vi "dfd_Create XML String for Subband Filters.vi"(7 "Bank":enum16{"AnalysisBank", "SynthesisBank"}(ring), 11 "filters":T1[](array[typedef]) {"mMRate_SumWl" min=1 max=32 step=1; "mMRate_InputIwl" min=1 max=32 step=1; "mMRate_GainWl" min=1 max=32 step=1; "mMRate_OutputWl" min=1 max=32 step=1; "mMRate_InputWl" min=1 max=32 step=1; "mMRate_CoefWl" min=1 max=32 step=1; "mMRate_Mode" items=["Default"=-1, "No Rate Change"=0, "Interpolation"=1, "Decimation"=2, "Interpolated"=3, "Rational"=4]}) -> (3 "xml string out":string)   [LabVIEW 2017, in "NI_DigFilter_FilterBank.lvlib"]
uses:
  <vilib>/addons/Digital Filter Design/NI_DigFilter_FilterBank.lvlib
  <vilib>/addons/Digital Filter Design/_Objects.llb/DFD Multirate Filter Obj.ctl
  <vilib>/addons/Digital Filter Design/_Objects.llb/DFD Multirate Mode.ctl
  <vilib>/addons/Digital Filter Design/_Objects.llb/DFD Coef Norm Type.ctl
  <vilib>/addons/Digital Filter Design/_Objects.llb/DFD Round-off Mode.ctl
  <vilib>/addons/Digital Filter Design/_Objects.llb/DFD FXP MRate Multiply Mode.ctl
  <vilib>/addons/Digital Filter Design/NI_DigFilter_Process.lvlib
  <vilib>/addons/Digital Filter Design/NI_DigFilterLicensed.lvlib
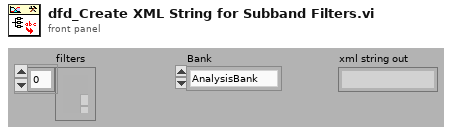
[diagram p1: front panel]
types:
  T1 = typedef "NI_DigFilterLicensed.lvlib/DFD Multirate Filter Obj.ctl" = cluster{"mMRate_Structure":enum16{"CIC", "FIR", "IIR", "Lattice"}, "mMRate_Mode":T2, "mMRate_Factor":i32, "mMRate_FIRParams":cluster{"mMRate_FIR_H":dbl[], "mMRate_FIR_IsNyquist?":bool, "mMRate_FIR_IsSymmetric?":bool}, "mMRate_CICParams":cluster{"mMRate_CIC_#Stage":i32, "mMRate_CIC_Lag":i32, "mMRate_CIC_Type":enum16{"Lowpass", "Highpass"}}, "mMRate_Order":i32, "mMRate_Version":string, "mMRate_Comments":string, "mMRate_RationalFactor":cluster{"mMRate_L":i32, "mMRate_M":i32}, "mMRate_Fs":dbl, "mMRate_Quantized?":bool, "mMRate_QFilterGain":dbl, "mMRate_CoefWl":i16, "mMRate_Scaling":cluster{"mMRate_ScaleByPowerOf2?":bool, "mMRate_ScaleType":T3}, "mMRate_InputWl":i16, "mMRate_OutputWl":i16, "mMRate_OutputMode":T4, "mMRate_MultMode":T5, "mMRate_BitPruning":bool, "mMRate_GainWl":i16, "mMRate_OutputFwl":i16, "mMRate_SumIwl":i16, "mMRate_InputIwl ":i16, "mMRate_SumWl":i16, "mMRate_CoefIwl":i16}
  T2 = typedef "NI_DigFilterLicensed.lvlib/DFD Multirate Mode.ctl" = i16
  T3 = typedef "NI_DigFilterLicensed.lvlib/DFD Coef Norm Type.ctl" = enum16{"No Norm", "Time Domain 1-Norm", "Time Domain 2-Norm", "Time Domain Inf-Norm"}
  T4 = typedef "NI_DigFilterLicensed.lvlib/DFD Round-off Mode.ctl" = enum16{"Nearest", "Truncation"}
  T5 = typedef "NI_DigFilterLicensed.lvlib/DFD FXP MRate Multiply Mode.ctl" = enum16{"Truncated", "Full"}
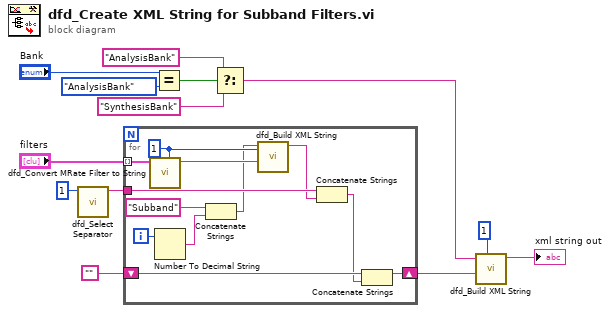
[diagram p0: block diagram]
diagram:
  n1 = call <vilib>:"dfd_Select Separator.vi"("indent order"=1) -> ("separator"=w11:string)  [unwired: 10 out]
  n2 = for {
    tunnel: "filters" -> [w25] mode=indexing
    tunnel: w11 -> [w24]
    shift-right: [w15] -> w12
    shift-left: "" -> [w16]
    i -> [w23]
    w22 = 1 ("indent order")
    n3 = call <vilib>:"dfd_Convert MRate Filter to String.vi"("indent order"=w22, "multirate filter in"=w25) -> ("xml string"=w20:string)  [unwired: 1 in, 8 out]
    n4 = Number To Decimal String(number=w23) -> (decimal integer string=w18:string)  [unwired: 1 out]
    n5 = Concatenate Strings("Subband" ("string"), w18) -> (w17:string)
    n6 = call <vilib>:"dfd_Build XML String.vi"("indent order"=w22, "string in"=w20, "element name"=w17) -> ("xml string out"=w21:string)  [unwired: 1 in, 7 out]
    n7 = Concatenate Strings(w24, w21) -> (w14:string)
    n8 = Concatenate Strings(w16, w14) -> (w15:string)
  }
  n9 = Equal?(x="Bank", y=enum16{"AnalysisBank", "SynthesisBank"}."AnalysisBank") -> (x = y?=w5:bool)
  n10 = Select(t="AnalysisBank" ("string"), s=w5, f="SynthesisBank" ("string")) -> (s? t:f=w2:string)
  n11 = call <vilib>:"dfd_Build XML String.vi"("indent order"=1, "string in"=w12, "element name"=w2) -> ("xml string out"=→"xml string out":string)  [unwired: 1 in, 7 out]
